vi "MNK_FP to PGSQL.vi"(8 "error in (no error)":errorcluster, 10 "str":string[](array[string]), 11 "dbl":dbl[](array[numeric])) -> (0 "error out":errorcluster)   [LabVIEW 2013]
uses:
  shared/postgreSQL-lv/Data.PG/Data.PGSQL.lvclass
panel:
  # "MNK FP to PGSQL"
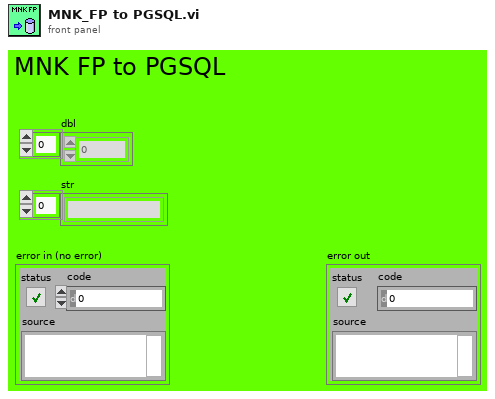
[diagram p1: front panel]
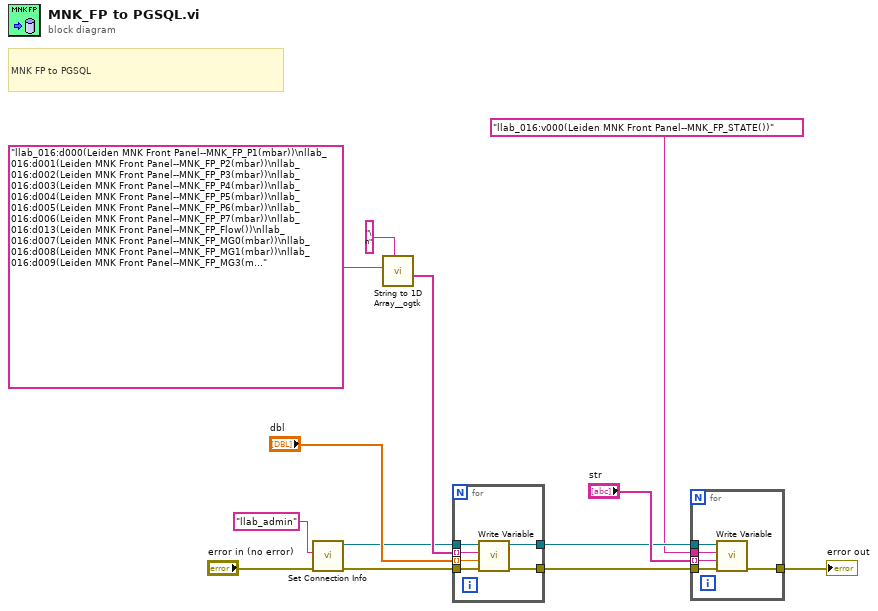
[diagram p0: block diagram]
diagram:
  # "MNK FP to PGSQL"
  n1 = call "Set Connection Info.vi"("username"="llab_admin", "error in (no error)"="error in (no error)") -> ("Data.PG out"=w5:refnum<class "Data.PGSQL.lvclass">, "error out"=w4:errorcluster)  [unwired: 7 in]
  n2 = call <userlib>:"String to 1D Array__ogtk.vi"("delimiter (Tab)"="\n", "string"="llab_016:d000(Leiden MNK Front Panel--MNK_FP_P1(mbar))\nllab_016:d001(Leiden MNK Front Panel--MNK_FP_P2(mbar))\nllab_016:d002(Leiden MNK Front Panel--MNK_FP_P3(mbar))\nllab_016:d003(Leiden MNK Front Panel--MNK_FP_P4(mbar))\nllab_016:d004(Leiden MNK Front Panel--MNK_FP_P5(mbar))\nllab_016:d005(Leiden MNK Front Panel--MNK_FP_P6(mbar))\nllab_016:d006(Leiden MNK Front Panel--MNK_FP_P7(mbar))\nllab_016:d013(Leiden MNK Front Panel--MNK_FP_Flow())\nllab_016:d007(Leiden MNK Front Panel--MNK_FP_MG0(mbar))\nllab_016:d008(Leiden MNK Front Panel--MNK_FP_MG1(mbar))\nllab_016:d009(Leiden MNK Front Panel--MNK_FP_MG3(mbar))\nllab_016:d010(Leiden MNK Front Panel--MNK_FP_MG4(mbar))\nllab_016:d011(Leiden MNK Front Panel--MNK_FP_MG5(mbar))\nllab_016:d014(Leiden MNK Front Panel--MNK_FP_state0())\nllab_016:d015(Leiden MNK Front Panel--MNK_FP_state1())\nllab_016:d016(Leiden MNK Front Panel--MNK_FP_state2())") -> ("Array of Strings"=w9:string[])  [unwired: 9 in]
  n3 = for {
    tunnel: w4 -> [w19]
    tunnel: w5 -> [w18]
    tunnel: w9 -> [w17] mode=indexing
    tunnel: [w16] -> w3
    tunnel: [w15] -> w6
    tunnel: "dbl" -> [w14] mode=indexing
    n4 = call "Write Variable.vi"("error in (no error)"=w19, "Data"=w14, "variable"=w17, "Data.PG in"=w18) -> ("error out"=w16:errorcluster, "Data.PG out"=w15:refnum<class "Data.PGSQL.lvclass">)  [unwired: 5 in, 1 out]
  }
  n5 = for {
    tunnel: w3 -> [w24]
    tunnel: w6 -> [w23]
    tunnel: [w22] -> w1
    tunnel: "llab_016:v000(Leiden MNK Front Panel--MNK_FP_STATE())" -> [w21]
    tunnel: "str" -> [w20] mode=indexing
    n6 = call "Write Variable.vi"("error in (no error)"=w24, "Data"=w20, "variable"=w21, "Data.PG in"=w23) -> ("error out"=w22:errorcluster)  [unwired: 5 in, 2 out]
  }
  "error out" <- w1
